vi "CAN Initialize FD.vi"(8 "error in (no error)":errorcluster, 10 "BitrateFD":string, 11 "Channel":u16) -> (0 "error out":errorcluster, 2 "BitrateFD out":string, 3 "function return":u32)   [LabVIEW 2025, in "PCAN2023.lvlib"]
doc: "Initializes a FD capable PCAN Channel\n\n\nTPCANStatus __stdcall CAN_InitializeFD(\n TPCANHandle Channel,\n TPCANBitrateFD BitrateFD);"
uses:
  PCAN2023.lvlib
  PCANBasic.dll
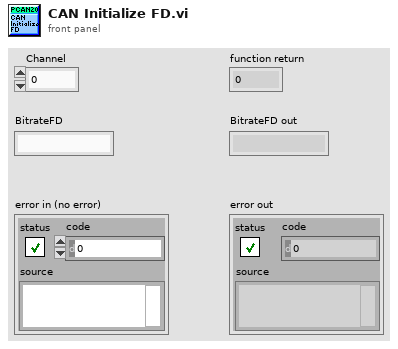
[diagram p1: front panel]
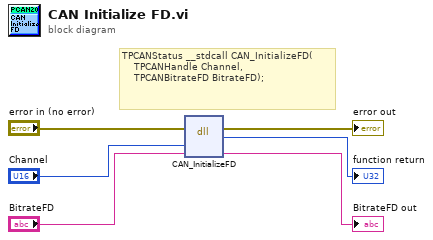
[diagram p0: block diagram]
diagram:
  # "TPCANStatus __stdcall CAN_InitializeFD(\n    TPCANHandle Channel,\n    TPCANBitrateFD BitrateFD);"
  n1 = dll-call lib="PCANBasic.*" fn="CAN_InitializeFD"(error in="error in (no error)", "Channel"="Channel", "BitrateFD"="BitrateFD") -> (error out=→"error out":errorcluster, →"function return":u32, "BitrateFD"=→"BitrateFD out":string)  [unwired: 3 in, 1 out]
